vi "PicoScope3000aStartStreaming.vi"(0 "error in":errorcluster, 3 "handle in":i16=1, 4 "Acquisition Settings":T1={"Auto Stop"=TRUE, "Desired Sample Interval"=1, "Pre-trigger Samples"=0, "Post-trigger Samples"=1000000, "Down-Sample Ratio"=1, "Down-Sample Mode"=0, "Overview Buffer Size"=100000, "Time Units"=3, "Four Channel Device?"=FALSE} {"Time Units" items=["Nanoseconds (ns)"=2, "Microseconds (us)"=3, "Milliseconds (ms)"=4, "Seconds (s)"=5]; "Down-Sample Mode" items=["None"=0, "Aggregate"=1, "Decimate"=2, "Average"=4]}, 5 "deviceIndex":u16, 7 "Enabled Array":i16[](array[numeric]), 21 "MSO Device?":bool) -> (8 "Channel A":i16[](array[numeric]), 9 "Channel C":i16[](array[numeric]), 10 "Channel A Min":i16[](array[numeric]), 11 "Channel C Min":i16[](array[numeric]), 12 "Channel B":i16[](array[numeric]), 13 "Channel D":i16[](array[numeric]), 14 "Channel B Min":i16[](array[numeric]), 15 "Channel D Min":i16[](array[numeric]), 16 "Port 0":i16[](array[numeric]), 17 "Port 1":i16[](array[numeric]), 18 "Port 0 Min":i16[](array[numeric]), 19 "Port 1 Min":i16[](array[numeric]), 20 "error out":errorcluster, 23 "handle out":i16=1, 24 "Sample Interval":u32=1000, 25 "sampleIntervalTimeUnits":i32)   [LabVIEW 2016]
doc: "This VI starts the oscilloscope streaming. It outputs arrays that will contain samples once PicoScope3000aGetStreamingValues.vi has returned."
uses:
  ps3000a.dll
  ps3000aWrap.dll
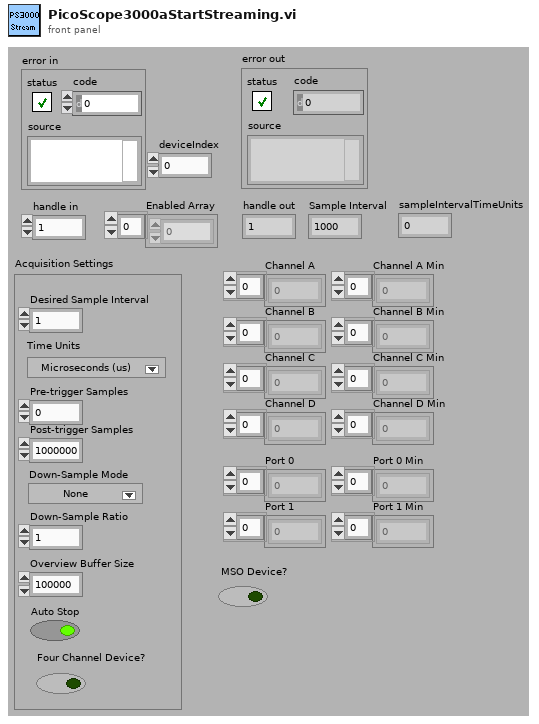
[diagram p1: front panel]
types:
  T1 = cluster{"Auto Stop":bool, "Desired Sample Interval":u32, "Pre-trigger Samples":u32, "Post-trigger Samples":u32, "Down-Sample Ratio":u32, "Down-Sample Mode":i32, "Overview Buffer Size":u32, "Time Units":u32, "Four Channel Device?":bool}
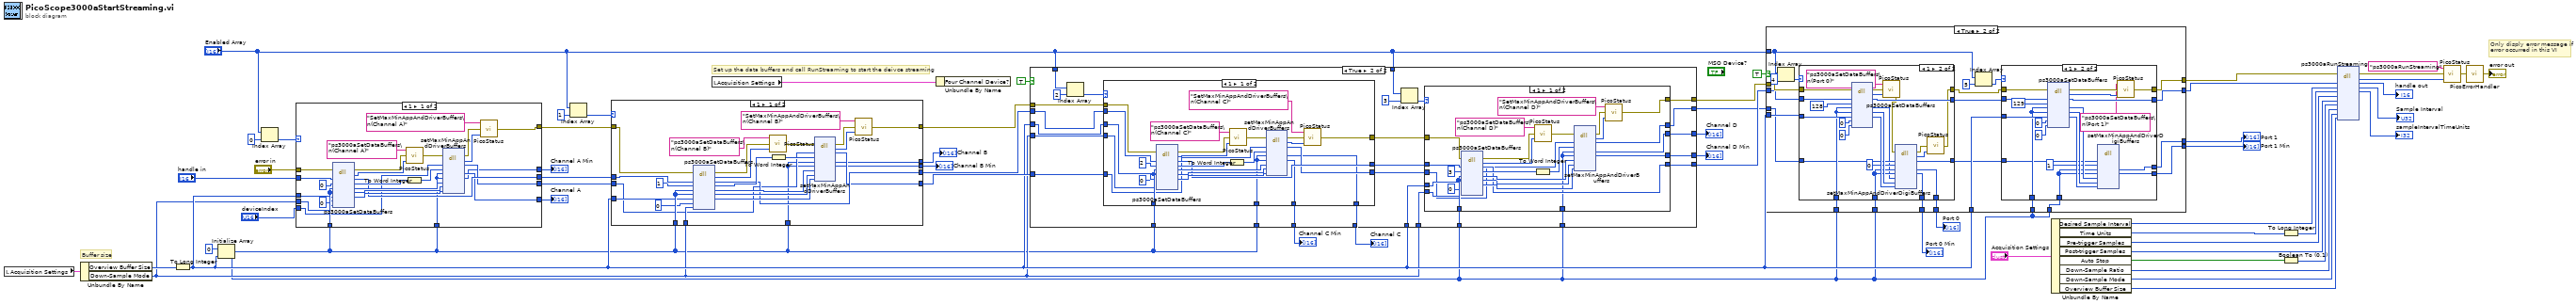
[diagram p0: block diagram]
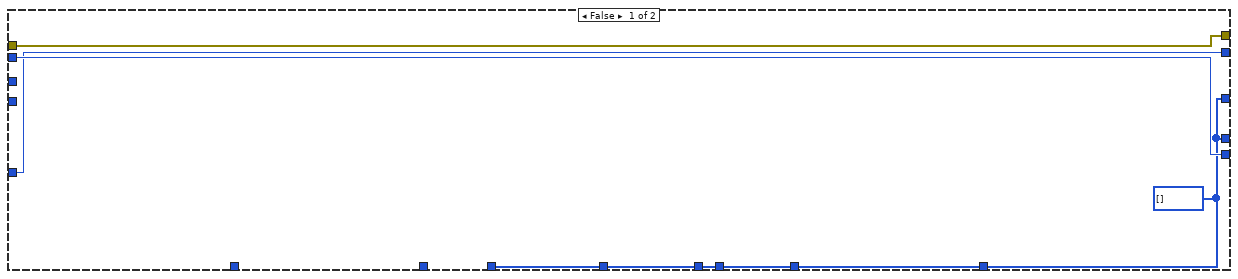
[diagram p2: hidden frame]
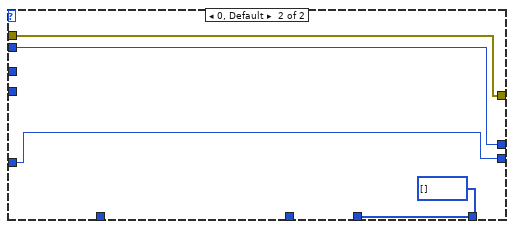
[diagram p3: hidden frame]
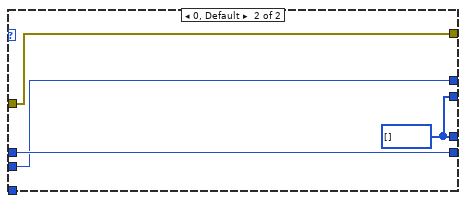
[diagram p4: hidden frame]
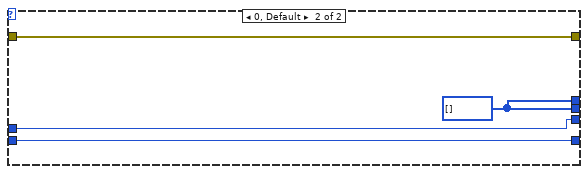
[diagram p5: hidden frame]
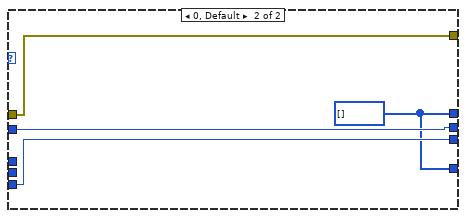
[diagram p6: hidden frame]
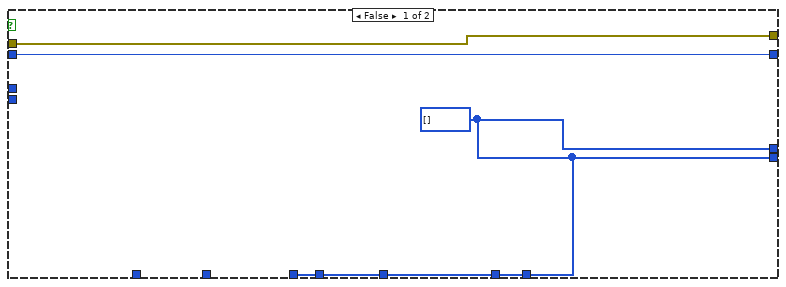
[diagram p7: hidden frame]
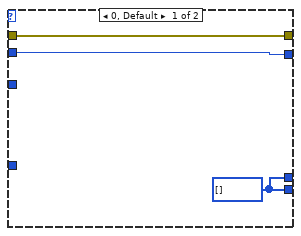
[diagram p8: hidden frame]
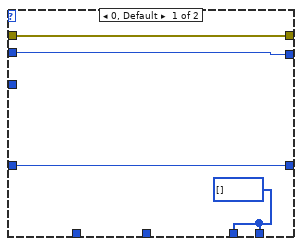
[diagram p9: hidden frame]
diagram:
  # "Only disply error message if\nerror occurred in this VI"
  # "Buffer size"
  # "Set up the data buffers and call RunStreaming to start the deivce streaming"
  n1 = local read "Acquisition Settings"() -> (w45:T1)
  n2 = Unbundle By Name(w45) -> ("Overview Buffer Size"=w13:u32, "Down-Sample Mode"=w7:i32)
  n3 = To Long Integer(number=w13) -> (32bit integer=w12:i32)
  n4 = Initialize Array(i16 0 ("element"), w12) -> (w4:i16[])
  n5 = Index Array(array="Enabled Array", index=0) -> (element=w35:i16)
  n6 = case shown="1" w35 {
    tunnel: "error in" -> [w85 w89]
    tunnel: [w67 w89] -> w28
    tunnel: "handle in" -> [w84 w88]
    tunnel: w4 -> [w82 _]
    tunnel: w12 -> [w81 _]
    tunnel: [w74 w88] -> w26
    tunnel: "deviceIndex" -> [w73 w87]
    tunnel: [w72 w87] -> w25
    tunnel: [w63 w86] -> w31
    tunnel: [w62 w86] -> w30
    tunnel: w4 -> [w61 _]
    tunnel: w7 -> [w60 _]
    frame 1 {
      n7 = dll-call lib="ps3000a.dll" fn="ps3000aSetDataBuffers" ("ps3000.dll:_ps3000_open_unit@0")(error in=w85, "handle"=w84, "channel"=0, "bufferMax"=w82, "bufferMin"=w82, "bufferLth"=w81, "segmentIndex"=u32 0, "mode"=w60) -> (error out=w70:errorcluster, "PICO_STATUS"=w69:u32, "handle"=w74:i16, "channel"=w76:i32, "bufferMax"=w78:i16[], "bufferMin"=w77:i16[], "bufferLth"=w79:i32)  [unwired: 4 in, 1 out]
      n8 = To Word Integer(number=w76) -> (16bit integer=w75:i16)
      n9 = call "PicoStatus.vi"("PICO STATUS"=w69, "error in"=w70, "source"="ps3000aSetDataBuffers\n(Channel A)") -> ("error out"=w71:errorcluster)
      n10 = dll-call lib="ps3000aWrap.dll" fn="setMaxMinAppAndDriverBuffers"(error in=w71, "deviceIndex"=w73, "channel"=w75, "appMaxBuffer"=w61, "appMinBuffer"=w61, "driverMaxBuffer"=w78, "driverMinBuffer"=w77, "bufferLenght"=w79) -> (error out=w66:errorcluster, "Pico Status"=w65:u32, "deviceIndex"=w72:u16, "appMaxBuffer"=w63:i16[], "appMinBuffer"=w62:i16[])  [unwired: 6 in, 1 out]
      n11 = call "PicoStatus.vi"("PICO STATUS"=w65, "error in"=w66, "source"="SetMaxMinAppAndDriverBuffers\n(Channel A)") -> ("error out"=w67:errorcluster)
    }
    frame 0, Default {
      w86 = i16[] [] ("appMinBuffer")
    }
  }
  "Channel A" <- w31
  "Channel A Min" <- w30
  n12 = Index Array(array="Enabled Array", index=1) -> (element=w24:i16)
  n13 = case shown="1" w24 {
    tunnel: w28 -> [w115 w119]
    tunnel: [w96 w119] -> w29
    tunnel: w26 -> [w114 w118]
    tunnel: w4 -> [w112 _]
    tunnel: w12 -> [w111 _]
    tunnel: w7 -> [w109 _]
    tunnel: [w103 w118] -> w20
    tunnel: w25 -> [w102 w117]
    tunnel: [w101 w117] -> w21
    tunnel: [w92 w116] -> w19
    tunnel: [w91 w116] -> w18
    tunnel: w4 -> [w90 _]
    frame 1 {
      n14 = dll-call lib="ps3000a.dll" fn="ps3000aSetDataBuffers" ("ps3000.dll:_ps3000_open_unit@0")(error in=w115, "handle"=w114, "channel"=1, "bufferMax"=w112, "bufferMin"=w112, "bufferLth"=w111, "segmentIndex"=u32 0, "mode"=w109) -> (error out=w99:errorcluster, "PICO_STATUS"=w98:u32, "handle"=w103:i16, "channel"=w105:i32, "bufferMax"=w107:i16[], "bufferMin"=w106:i16[], "bufferLth"=w108:i32)  [unwired: 4 in, 1 out]
      n15 = call "PicoStatus.vi"("PICO STATUS"=w98, "error in"=w99, "source"="ps3000aSetDataBuffers\n(Channel B)") -> ("error out"=w100:errorcluster)
      n16 = To Word Integer(number=w105) -> (16bit integer=w104:i16)
      n17 = dll-call lib="ps3000aWrap.dll" fn="setMaxMinAppAndDriverBuffers"(error in=w100, "deviceIndex"=w102, "channel"=w104, "appMaxBuffer"=w90, "appMinBuffer"=w90, "driverMaxBuffer"=w107, "driverMinBuffer"=w106, "bufferLenght"=w108) -> (error out=w95:errorcluster, "Pico Status"=w94:u32, "deviceIndex"=w101:u16, "appMaxBuffer"=w92:i16[], "appMinBuffer"=w91:i16[])  [unwired: 6 in, 1 out]
      n18 = call "PicoStatus.vi"("PICO STATUS"=w94, "error in"=w95, "source"="SetMaxMinAppAndDriverBuffers\n(Channel B)") -> ("error out"=w96:errorcluster)
    }
    frame 0, Default {
      w116 = i16[] [] ("appMaxBuffer")
    }
  }
  "Channel B" <- w19
  "Channel B Min" <- w18
  n19 = local read "Acquisition Settings"() -> (w50:T1)
  n20 = Unbundle By Name(w50) -> ()  [unwired: 1 out]
  n21 = case shown="True" TRUE {
    tunnel: w29 -> [w123 w150]
    tunnel: [w123 w148] -> w27
    tunnel: [w122 w147] -> w22
    tunnel: "Enabled Array" -> [_ w143]
    tunnel: w4 -> [_ w141]
    tunnel: w4 -> [_ w140]
    tunnel: w21 -> [w120 w139]
    tunnel: w20 -> [w122 w137]
    tunnel: w4 -> [_ w135]
    tunnel: w4 -> [_ w134]
    tunnel: w12 -> [_ w133]
    tunnel: w7 -> [_ w132]
    tunnel: w12 -> [_ w131]
    tunnel: [w121 w130] -> w17
    tunnel: [w121 w129] -> w16
    tunnel: [w121 w128] -> w15
    tunnel: [w121 w127] -> w14
    tunnel: "Enabled Array" -> [_ w126]
    tunnel: w7 -> [_ w125]
    tunnel: [w120 w124] -> w6
    frame False {
      w121 = i16[] [] ("appMaxBuffer")
    }
    frame True {
      n22 = Index Array(array=w143, index=2) -> (element=w145:i16)
      n23 = case shown="1" w145 {
        tunnel: w150 -> [w176 w180]
        tunnel: [w157 w180] -> w149
        tunnel: w137 -> [w175 w179]
        tunnel: w141 -> [w173 _]
        tunnel: w131 -> [w172 _]
        tunnel: w132 -> [w170 _]
        tunnel: [w164 w179] -> w136
        tunnel: w139 -> [w163 w178]
        tunnel: [w162 w178] -> w138
        tunnel: [w153 w177] -> w130
        tunnel: [w152 w177] -> w129
        tunnel: w140 -> [w151 _]
        frame 1 {
          n24 = dll-call lib="ps3000a.dll" fn="ps3000aSetDataBuffers" ("ps3000.dll:_ps3000_open_unit@0")(error in=w176, "handle"=w175, "channel"=2, "bufferMax"=w173, "bufferMin"=w173, "bufferLth"=w172, "segmentIndex"=u32 0, "mode"=w170) -> (error out=w160:errorcluster, "PICO_STATUS"=w159:u32, "handle"=w164:i16, "channel"=w166:i32, "bufferMax"=w168:i16[], "bufferMin"=w167:i16[], "bufferLth"=w169:i32)  [unwired: 4 in, 1 out]
          n25 = To Word Integer(number=w166) -> (16bit integer=w165:i16)
          n26 = call "PicoStatus.vi"("PICO STATUS"=w159, "error in"=w160, "source"="ps3000aSetDataBuffers\n(Channel C)") -> ("error out"=w161:errorcluster)
          n27 = dll-call lib="ps3000aWrap.dll" fn="setMaxMinAppAndDriverBuffers"(error in=w161, "deviceIndex"=w163, "channel"=w165, "appMaxBuffer"=w151, "appMinBuffer"=w151, "driverMaxBuffer"=w168, "driverMinBuffer"=w167, "bufferLenght"=w169) -> (error out=w156:errorcluster, "Pico Status"=w155:u32, "deviceIndex"=w162:u16, "appMaxBuffer"=w153:i16[], "appMinBuffer"=w152:i16[])  [unwired: 6 in, 1 out]
          n28 = call "PicoStatus.vi"("PICO STATUS"=w155, "error in"=w156, "source"="SetMaxMinAppAndDriverBuffers\n(Channel C)") -> ("error out"=w157:errorcluster)
        }
        frame 0, Default {
          w177 = i16[] [] ("appMinBuffer")
        }
      }
      n29 = Index Array(array=w126, index=3) -> (element=w144:i16)
      n30 = case shown="1" w144 {
        tunnel: w149 -> [w206 w210]
        tunnel: [w187 w210] -> w148
        tunnel: w136 -> [w205 w209]
        tunnel: w135 -> [w203 _]
        tunnel: w133 -> [w202 _]
        tunnel: w125 -> [w200 _]
        tunnel: [w194 w209] -> w147
        tunnel: w138 -> [w193 w208]
        tunnel: [w192 w208] -> w124
        tunnel: [w183 w207] -> w128
        tunnel: [w182 w207] -> w127
        tunnel: w134 -> [w181 _]
        frame 1 {
          n31 = dll-call lib="ps3000a.dll" fn="ps3000aSetDataBuffers" ("ps3000.dll:_ps3000_open_unit@0")(error in=w206, "handle"=w205, "channel"=3, "bufferMax"=w203, "bufferMin"=w203, "bufferLth"=w202, "segmentIndex"=u32 0, "mode"=w200) -> (error out=w190:errorcluster, "PICO_STATUS"=w189:u32, "handle"=w194:i16, "channel"=w196:i32, "bufferMax"=w198:i16[], "bufferMin"=w197:i16[], "bufferLth"=w199:i32)  [unwired: 4 in, 1 out]
          n32 = To Word Integer(number=w196) -> (16bit integer=w195:i16)
          n33 = call "PicoStatus.vi"("PICO STATUS"=w189, "error in"=w190, "source"="ps3000aSetDataBuffers\n(Channel D)") -> ("error out"=w191:errorcluster)
          n34 = dll-call lib="ps3000aWrap.dll" fn="setMaxMinAppAndDriverBuffers"(error in=w191, "deviceIndex"=w193, "channel"=w195, "appMaxBuffer"=w181, "appMinBuffer"=w181, "driverMaxBuffer"=w198, "driverMinBuffer"=w197, "bufferLenght"=w199) -> (error out=w186:errorcluster, "Pico Status"=w185:u32, "deviceIndex"=w192:u16, "appMaxBuffer"=w183:i16[], "appMinBuffer"=w182:i16[])  [unwired: 6 in, 1 out]
          n35 = call "PicoStatus.vi"("PICO STATUS"=w185, "error in"=w186, "source"="SetMaxMinAppAndDriverBuffers\n(Channel D)") -> ("error out"=w187:errorcluster)
        }
        frame 0, Default {
          w207 = i16[] [] ("appMinBuffer")
        }
      }
    }
  }
  "Channel C" <- w17
  "Channel D" <- w15
  "Channel C Min" <- w16
  "Channel D Min" <- w14
  n36 = case shown="True" TRUE {
    tunnel: w27 -> [w213 w236]
    tunnel: w22 -> [w212 w235]
    tunnel: w4 -> [_ w225]
    tunnel: w12 -> [_ w234]
    tunnel: w12 -> [_ w233]
    tunnel: [w211 w218] -> w43
    tunnel: [w211 w217] -> w41
    tunnel: [w211 w232] -> w42
    tunnel: [w212 w230] -> w40
    tunnel: [w213 w229] -> w44
    tunnel: [w211 w227] -> w39
    tunnel: w4 -> [_ w226]
    tunnel: "Enabled Array" -> [_ w214]
    tunnel: w4 -> [_ w222]
    tunnel: w6 -> [_ w221]
    tunnel: w4 -> [_ w216]
    frame False {
      w211 = i16[] [] ("bufferMin")
    }
    frame True {
      n37 = Index Array(array=w214, index=4) -> (element=w223:i16)
      n38 = case shown="1" w223 {
        tunnel: w236 -> [w263 w287]
        tunnel: w235 -> [w262 w286]
        tunnel: w234 -> [_ w284]
        tunnel: [w261 w272] -> w217
        tunnel: [w261 w264] -> w218
        tunnel: [w263 w266] -> w231
        tunnel: [w262 w280] -> w228
        tunnel: w225 -> [_ w279]
        tunnel: w222 -> [_ w276]
        tunnel: w221 -> [w260 w273]
        tunnel: [w260 w271] -> w215
        frame 0, Default {
          w261 = i16[] [] ("bufferMin")
        }
        frame 1 {
          n39 = dll-call lib="ps3000a.dll" fn="ps3000aSetDataBuffers" ("ps3000.dll:_ps3000_open_unit@0")(error in=w287, "handle"=w286, "channel"=128, "bufferMax"=w279, "bufferMin"=w279, "bufferLth"=w284, "segmentIndex"=u32 0, "mode"=0) -> (error out=w274:errorcluster, "PICO_STATUS"=w281:u32, "handle"=w280:i16, "bufferMax"=w265:i16[], "bufferMin"=w278:i16[], "bufferLth"=w277:i32)  [unwired: 5 in, 1 out]
          n40 = call "PicoStatus.vi"("PICO STATUS"=w281, "error in"=w274, "source"="ps3000aSetDataBuffers\n(Port 0)") -> ("error out"=w270:errorcluster)
          n41 = dll-call lib="ps3000aWrap.dll" fn="setMaxMinAppAndDriverDigiBuffers"(error in=w270, "deviceIndex"=w273, "digiport"=i16 0, "appMaxDigiBuffer"=w276, "appMinDigiBuffer"=w276, "driverMaxDigiBuffer"=w265, "driverMinDigiBuffer"=w278, "bufferLength"=w277) -> (error out=w268:errorcluster, "PICO STATUS"=w267:u32, "deviceIndex"=w271:u16, "appMaxDigiBuffer"=w272:i16[], "appMinDigiBuffer"=w264:i16[])  [unwired: 6 in, 1 out]
          n42 = call "PicoStatus.vi"("PICO STATUS"=w267, "error in"=w268) -> ("error out"=w266:errorcluster)  [unwired: 1 in]
        }
      }
      n43 = Index Array(array=w214, index=5) -> (element=w220:i16)
      n44 = case shown="1" w220 {
        tunnel: w233 -> [_ w256]
        tunnel: [w237 w247] -> w232
        tunnel: w231 -> [w239 w253]
        tunnel: [w238 w252] -> w230
        tunnel: [w239 w251] -> w229
        tunnel: w228 -> [w238 w250]
        tunnel: [w237 w248] -> w227
        tunnel: w226 -> [_ w249]
        tunnel: w216 -> [_ w243]
        tunnel: w215 -> [_ w241]
        frame 0, Default {
          w237 = i16[] [] ("bufferMax")
        }
        frame 1 {
          n45 = dll-call lib="ps3000a.dll" fn="ps3000aSetDataBuffers" ("ps3000.dll:_ps3000_open_unit@0")(error in=w253, "handle"=w250, "channel"=129, "bufferMax"=w249, "bufferMin"=w249, "bufferLth"=w256, "segmentIndex"=u32 0, "mode"=0) -> (error out=w254:errorcluster, "PICO_STATUS"=w255:u32, "handle"=w252:i16, "bufferMax"=w246:i16[], "bufferMin"=w245:i16[], "bufferLth"=w244:i32)  [unwired: 5 in, 1 out]
          n46 = dll-call lib="ps3000aWrap.dll" fn="setMaxMinAppAndDriverDigiBuffers"("deviceIndex"=w241, "digiport"=i16 1, "appMaxDigiBuffer"=w243, "appMinDigiBuffer"=w243, "driverMaxDigiBuffer"=w246, "driverMinDigiBuffer"=w245, "bufferLength"=w244) -> ("appMaxDigiBuffer"=w248:i16[], "appMinDigiBuffer"=w247:i16[])  [unwired: 9 in, 2 out]
          n47 = call "PicoStatus.vi"("PICO STATUS"=w255, "error in"=w254, "source"="ps3000aSetDataBuffers\n(Port 1)") -> ("error out"=w251:errorcluster)
        }
      }
    }
  }
  "Port 0" <- w41
  "Port 1" <- w39
  "Port 1 Min" <- w42
  "Port 0 Min" <- w43
  n48 = Unbundle By Name("Acquisition Settings") -> ("Desired Sample Interval"=w10:u32, "Time Units"=w9:u32, "Pre-trigger Samples"=w53:u32, "Post-trigger Samples"=w52:u32, "Auto Stop"=w51:bool, "Down-Sample Ratio"=w47:u32, "Down-Sample Mode"=w46:i32, "Overview Buffer Size"=w11:u32)
  n49 = To Long Integer(number=w9) -> (32bit integer=w8:i32)
  n50 = Boolean To (0,1)(Boolean=w51) -> (0, 1=w54:i16)
  n51 = dll-call lib="ps3000a.dll" fn="ps3000aRunStreaming" ("ps3000.dll:_ps3000_open_unit@0")(error in=w44, "handle"=w40, "sampleInterval"=w10, "sampleIntervalTimeUnits"=w8, "PreTriggerSamples"=w53, "PostTriggerSamples"=w52, "autoStop"=w54, "downSampleRatio"=w47, "downSampleRatioMode"=w46, "overviewBufferSize"=w11) -> (error out=w57:errorcluster, "PICO_STATUS"=w58:u32, "handle"=→"handle out":i16, "sampleInterval"=→"Sample Interval":u32, "sampleIntervalTimeUnits"=→"sampleIntervalTimeUnits":i32)  [unwired: 8 in, 1 out]
  n52 = call "PicoStatus.vi"("PICO STATUS"=w58, "error in"=w57, "source"="ps3000aRunStreaming") -> ("error out"=w37:errorcluster)
  n53 = call "PicoErrorHandler.vi"("error in"=w37) -> ("error out"=→"error out":errorcluster)
